vi "Read Element of Q.vi"(8 "error in (no error)":errorcluster, 10 "indices":i32[](array[numeric]), 11 "Kalman Filter in":refnum<class "Kalman Filter.lvclass">) -> (0 "error out":errorcluster, 2 "Real Matrix Element":dbl, 3 "Kalman Filter out":refnum<class "Kalman Filter.lvclass">)   [LabVIEW 2014, in "Observer Library.lvlib" / "Kalman Filter.lvclass"]
uses:
  Kalman Filter.lvclass
  Kalman Filter.lvclass/Kalman Filter.ctl
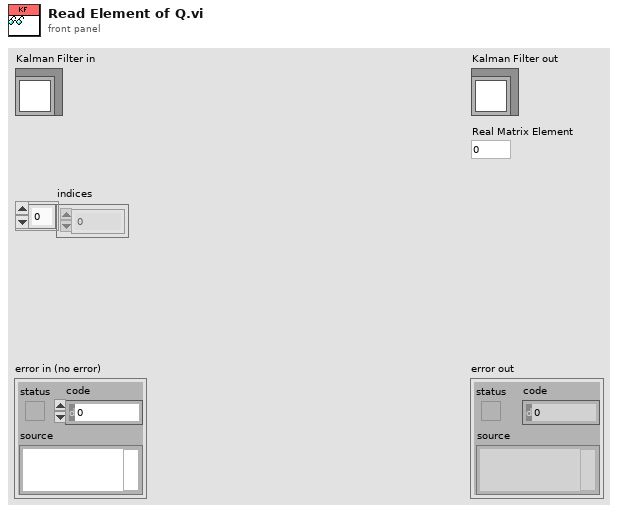
[diagram p1: front panel]
types:
  T1 = typedef "NI_Matrix.lvlib/RealMatrix.ctl" = dbl[][]
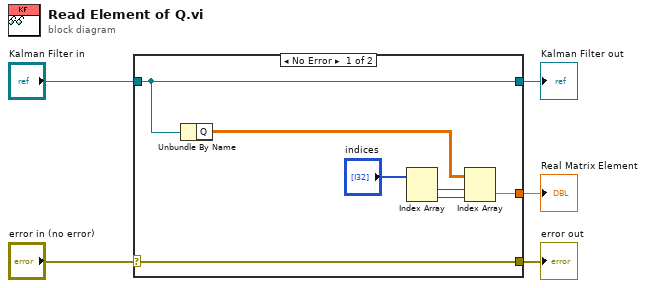
[diagram p0: block diagram]
diagram:
  n1 = case shown="No Error" "error in (no error)" {
    selector: "error in (no error)" -> [w12 w13]
    tunnel: [w12 w13] -> w4
    tunnel: [w11 w14] -> w2
    tunnel: "Kalman Filter in" -> [w11 w14]
    tunnel: [w10 _] -> w1
    frame No Error {
      n2 = Unbundle By Name(w11) -> ("Q"=w6:T1)
      n3 = Index Array(array="indices") -> (element #1=w8:i32, element #2=w7:i32)  [unwired: 2 in]
      n4 = Index Array(array=w6, index (row)=w8, index (col)=w7) -> (element=w10:dbl)
    }
    frame Error {
    }
  }
  "error out" <- w4
  "Kalman Filter out" <- w2
  "Real Matrix Element" <- w1
